vi "AnalogTrack.vi"(0 "controller in":refnum<k24>, 1 "axis name":string, 2 "analog output":i32, 3 "servo value":i32, 4 "scale factor":dbl=1.0, 5 "error in (no error)":errorcluster, 6 "offset value":dbl, 7 "return immediately":bool, 8 "min value":dbl, 10 "max value":dbl) -> (14 "controller out":refnum<k24>, 19 "error out":errorcluster)   [LabVIEW 2019]
uses:
  C:/Users/patrick/Documents/GitHub/Aerotech-Delay-Line/lvsrc/Aerotech-Ensemble-LabVIEW/2010-5.6/Bin/Aerotech.Ensemble.dll
  Bin/Aerotech.Ensemble.dll
  C:/Users/patrick/Documents/GitHub/Aerotech-Delay-Line/lvsrc/Aerotech-Ensemble-LabVIEW/2010-5.6/Bin/Aerotech.Ensemble.LabVIEW.dll
  Bin/Aerotech.Ensemble.LabVIEW.dll
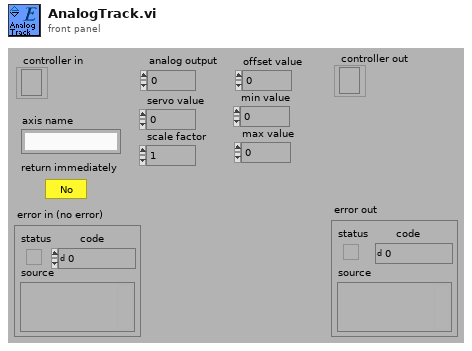
[diagram p1: front panel]
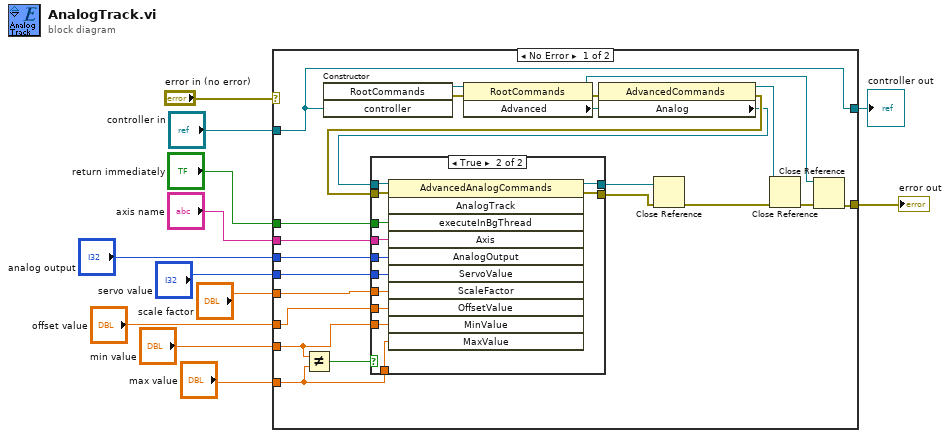
[diagram p0: block diagram]
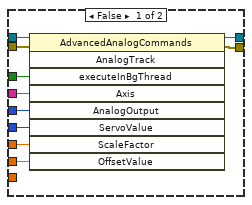
[diagram p2: hidden frame]
diagram:
  n1 = case shown="No Error" "error in (no error)" {
    selector: "error in (no error)" -> [_ w59]
    tunnel: [w31 w59] -> w11
    tunnel: "controller in" -> [w26 w58]
    tunnel: "return immediately" -> [w21 _]
    tunnel: "axis name" -> [w20 _]
    tunnel: "analog output" -> [w19 _]
    tunnel: [w26 w58] -> w7
    tunnel: "servo value" -> [w18 _]
    tunnel: "scale factor" -> [w17 _]
    tunnel: "offset value" -> [w16 _]
    tunnel: "min value" -> [w15 _]
    tunnel: "max value" -> [w14 _]
    frame No Error {
      n2 = Not Equal?(x=w15, y=w14) -> (x != y?=w13:bool)
      n3 = constructor class="RootCommands"("controller"=w26) -> (reference out=w35:refnum<k24>, error out=w34:errorcluster)  [unwired: 3 in, 2 out]
      n4 = property class="RootCommands"(reference=w35, error in=w34) -> (reference out=w28:refnum<k24>, error out=w33:errorcluster, "Advanced"=w32:refnum<k24>)
      n5 = property class="AdvancedCommands"(reference=w32, error in=w33) -> (reference out=w29:refnum<k24>, error out=w23:errorcluster, "Analog"=w22:refnum<k24>)
      n6 = case shown="True" w13 {
        tunnel: w22 -> [w45 w55]
        tunnel: w23 -> [w44 w54]
        tunnel: w21 -> [w43 w53]
        tunnel: w20 -> [w42 w52]
        tunnel: w19 -> [w41 w51]
        tunnel: [w40 w56] -> w25
        tunnel: [w39 w57] -> w24
        tunnel: w18 -> [w38 w50]
        tunnel: w17 -> [w37 w49]
        tunnel: w16 -> [w36 w48]
        tunnel: w15 -> [_ w47]
        tunnel: w14 -> [_ w46]
        frame False {
          n7 = invoke class="AdvancedAnalogCommands" method="AnalogTrack"(reference=w45, error in=w44, "executeInBgThread"=w43, "Axis"=w42, "AnalogOutput"=w41, "ServoValue"=w38, "ScaleFactor"=w37, "OffsetValue"=w36) -> (reference out=w39:refnum<k24>, error out=w40:errorcluster)  [unwired: 1 in, 7 out]
        }
        frame True {
          n8 = invoke class="AdvancedAnalogCommands" method="AnalogTrack"(reference=w55, error in=w54, "executeInBgThread"=w53, "Axis"=w52, "AnalogOutput"=w51, "ServoValue"=w50, "ScaleFactor"=w49, "OffsetValue"=w48, "MinValue"=w47, "MaxValue"=w46) -> (reference out=w57:refnum<k24>, error out=w56:errorcluster)  [unwired: 1 in, 9 out]
        }
      }
      n9 = Close Reference(reference=w24, error in (no error)=w25) -> (error out=w27:errorcluster)
      n10 = Close Reference(reference=w29, error in (no error)=w27) -> (error out=w30:errorcluster)
      n11 = Close Reference(reference=w28, error in (no error)=w30) -> (error out=w31:errorcluster)
    }
    frame Error {
    }
  }
  "error out" <- w11
  "controller out" <- w7
